vi "Add Receiver.vi"(8 "error in (no error)":errorcluster caption="错误输入（无错误）", 10 "Receiver Address":string, 11 "Email In":refnum<class "Email.lvclass"> caption="DNL_LabVIEW Object in") -> (0 "error out":errorcluster caption="错误输出", 3 "Email Out":refnum<class "Email.lvclass"> caption="DNL_LabVIEW Object out")   [LabVIEW 2012, in "Email.lvclass"]
uses:
  Email.lvclass
  Email.lvclass/Email.ctl
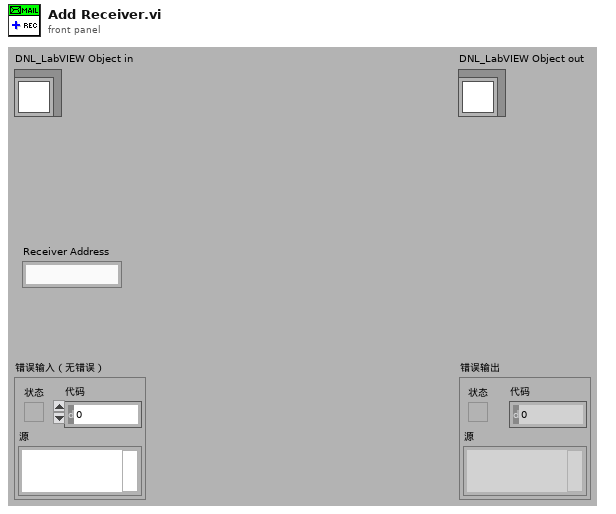
[diagram p1: front panel]
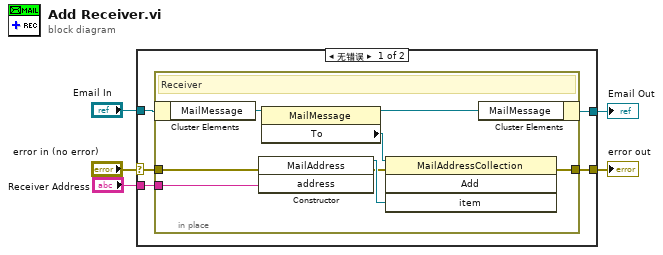
[diagram p0: block diagram]
diagram:
  n1 = case shown="无错误" "error in (no error)" {
    selector: "error in (no error)" -> [w8 w20]
    tunnel: [w7 w20] -> w4
    tunnel: [w6 w19] -> w2
    tunnel: "Email In" -> [w10 w19]
    tunnel: "Receiver Address" -> [w9 _]
    frame No Error {
      n2 = in-place {
        in-place-border: w9 -> [w14]
        in-place-border: w8 -> [w12]
        in-place-border: [w11] -> w7
        # "Receiver"
        n3 = in-place-cluster #1(w10) -> ("MailMessage"=w18:refnum<k24>)
        n4 = constructor class="MailAddress"(error in=w12, "address"=w14) -> (reference out=w15:refnum<k24>, error out=w13:errorcluster)  [unwired: 2 in, 2 out]
        n5 = property class="MailMessage"(reference=w18) -> (reference out=w16:refnum<k24>, "To"=w17:refnum<k24>)  [unwired: 1 in, 1 out]
        n6 = invoke class="MailAddressCollection" method="Add"(reference=w17, error in=w13, "item"=w15) -> (error out=w11:errorcluster)  [unwired: 1 in, 3 out]
        n7 = in-place-cluster #1("MailMessage"=w16) -> (w6:refnum<class "Email.lvclass">)
      }
    }
    frame Error {
    }
  }
  "error out" <- w4
  "Email Out" <- w2
